vi "AlliGator Check Gate Number in HDF5 File v2.vi"(7 "Gate Names":string[](array[string]), 8 "error in (no error)":errorcluster, 9 "FLI Parameters":T2, 11 "ref in":T1 format="%.0x") -> (0 "error out":errorcluster, 1 "FLI Parameters":T2, 3 "ref":T1 format="%.0x", 4 "Missing Gates?":bool, 6 "Additional Gates?":bool)   [LabVIEW 2021, in "AlliGator HDF5.lvlib"]
doc: "Checks that the gate images stored in the HDF5 file correspond to the description provided by the <B>FLI Parameters</B>.\n\nIf so updates <B># Gates</B> in that structure and sets the corresponding output flags."
uses:
  AlliGator HDF5.lvlib
  Phasor/Phasor Fluorescence Lifetime Parameters v2.ctl
  <vilib>/addons/h5labview2/base/hid_t.ctl
  Arrays/Linear Ramp End Options.ctl
  3b143c5f-f340-4cb5-b493-7761f7e72ec4.vi
  57e33c98-4f83-48b5-b2ca-9a3f9f880677.vi
  <userlib>/_OpenG.lib/array/array.llb/Filter 1D Array (I32)__ogtk.vi
  <vilib>/addons/h5labview2/group/H5G.lvlib
  Arrays/Arrays.lvlib
  <userlib>/_OpenG.lib/array/array.llb/openg_array.lvlib
  Phasor/Phasor.lvlib
panel:
  # "see the AlliGator License on the block diagram (Ctrl+E or Window:Show Block Diagram)"
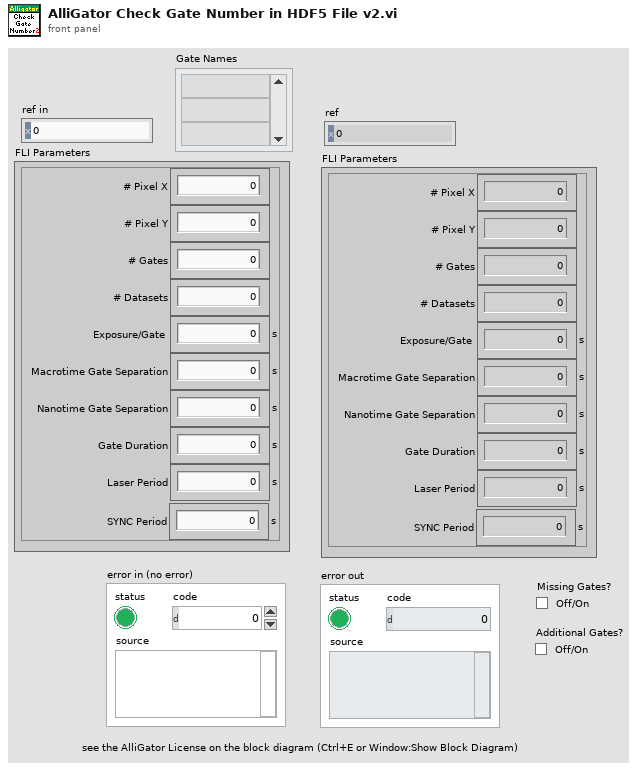
[diagram p1: front panel]
types:
  T1 = typedef "hid_t.ctl" = i64
  T2 = typedef "Phasor.lvlib/Phasor Fluorescence Lifetime Parameters v2.ctl" = cluster{"# Pixel X":i32, "# Pixel Y":i32, "# Gates":i32, "# Datasets":i32, "Exposure/Gate":dbl[unit], "Macrotime Gate Separation":dbl[unit], "Nanotime Gate Separation":dbl[unit], "Gate Duration":dbl[unit], "Laser Period":dbl[unit], "SYNC Period":dbl[unit]}
  T3 = typedef "Arrays.lvlib/Linear Ramp End Options.ctl" = enum16{"Include Min/Exclude Max", "Exclude Min/Include Max", "Include Both Ends", "Exclude Both Ends"}
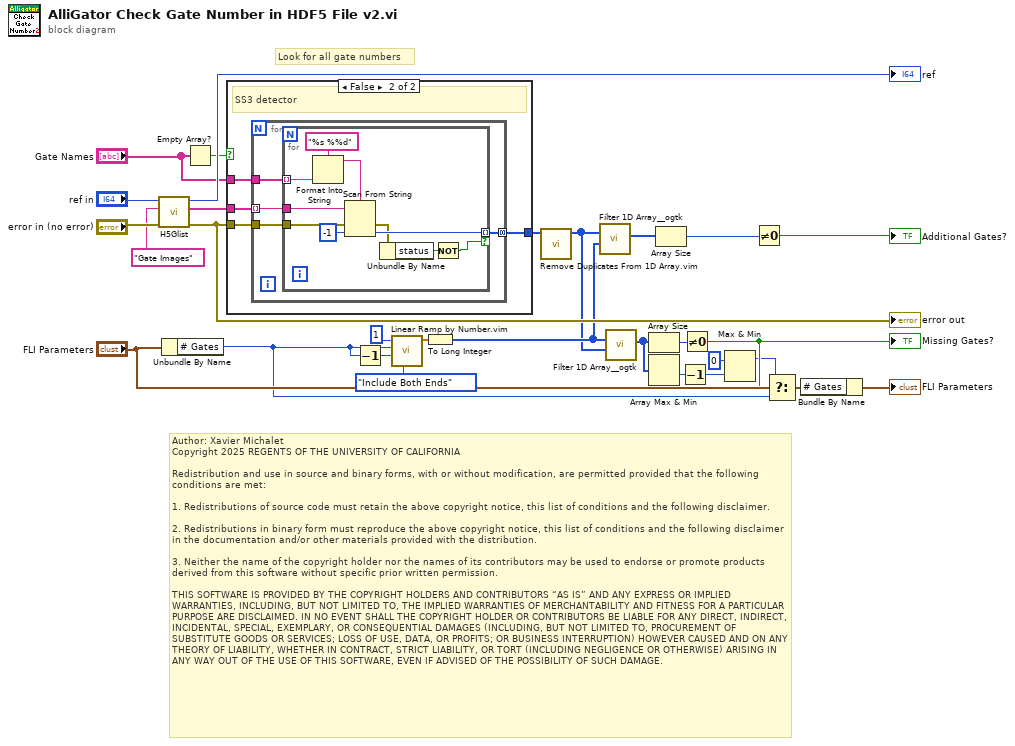
[diagram p0: block diagram]
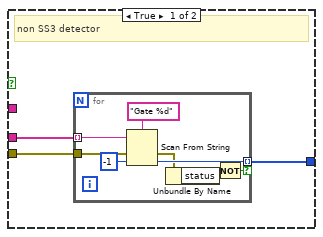
[diagram p2: hidden frame]
diagram:
  # "Author: Xavier Michalet\nCopyright 2025 REGENTS OF THE UNIVERSITY OF CALIFORNIA\n\nRedistribution and use in source and binary forms, with or without modification, are permitted provided that the following conditions are met:\n\n1. Redistributions of source code must retain the above copyright notice, this list of conditions and the following disclaimer.\n\n2. Redistributions in binary form must reproduce the above copyright notice, this list of conditions and the following disclaimer in the documentation and/or other materials provided with the distribution.\n\n3. Neither the name of the copyright holder nor the names of its contributors may be used to endorse or promote products derived from this software without specific prior written permission.\n\nTHIS SOFTWARE IS PROVIDED BY THE COPYRIGHT HOLDERS AND CONTRIBUTORS “AS IS” AND ANY EXPRESS OR IMPLIED WARRANTIES, INCLUDING, BUT NOT LIMITED TO, THE IMPLIED WARRANTIES OF MERCHANTABILITY AND FITNESS FOR A PARTICULAR PURPOSE ARE DISCLAIMED. IN NO EVENT SHALL THE COPYRIGHT HOLDER OR CONTRIBUTORS BE LIABLE FOR ANY DIRECT, INDIRECT, INCIDENTAL, SPECIAL, EXEMPLARY, OR CONSEQUENTIAL DAMAGES (INCLUDING, BUT NOT LIMITED TO, PROCUREMENT OF SUBSTITUTE GOODS OR SERVICES; LOSS OF USE, DATA, OR PROFITS; OR BUSINESS INTERRUPTION) HOWEVER CAUSED AND ON ANY THEORY OF LIABILITY, WHETHER IN CONTRACT, STRICT LIABILITY, OR TORT (INCLUDING NEGLIGENCE OR OTHERWISE) ARISING IN ANY WAY OUT OF THE USE OF THIS SOFTWARE, EVEN IF ADVISED OF THE POSSIBILITY OF SUCH DAMAGE."
  # "Look for all gate numbers"
  n1 = call <vilib>:"H5Glist.vi"("error in (no error)"="error in (no error)", "group (.)"="Gate Images" ("name"), "ref in"="ref in") -> ("error out"=w14:errorcluster, "names"=w23:string[], "ref out"=→"ref":T1)  [unwired: 5 in, 1 out]
  "error out" <- w14
  n2 = Unbundle By Name("FLI Parameters") -> ("# Gates"=w6:i32)
  n3 = Empty Array?(array="Gate Names") -> (empty?=w3:bool)
  n4 = case shown="False" w3 {
    tunnel: w23 -> [w32 w44]
    tunnel: [w31 w43] -> w19
    tunnel: w14 -> [w30 w42]
    tunnel: "Gate Names" -> [_ w41]
    frame True {
      # "non SS3 detector"
      n5 = for {
        tunnel: w32 -> [w39] mode=indexing
        tunnel: w30 -> [w38]
        tunnel: [w37] -> w31 mode=indexing if=w33
        n6 = Scan From String(format string="Gate %d" ("initial string"), input string=w39, error in=w38, default 1=-1 ("default value 1")) -> (error out=w36:errorcluster, output 1=w37:i32)  [unwired: 1 in, 2 out]
        n7 = Unbundle By Name(w36) -> ("status"=w35:bool)
        n8 = Not(x=w35) -> (.not. x?=w33:bool)
      }
    }
    frame False {
      # "SS3 detector"
      n9 = for {
        tunnel: w44 -> [w48] mode=indexing
        tunnel: w42 -> [w47]
        tunnel: [w46] -> w43 mode=concatenating
        tunnel: w41 -> [w45]
        n10 = for {
          tunnel: w48 -> [w58]
          tunnel: w47 -> [w57]
          tunnel: [w56] -> w46 mode=indexing if=w49
          tunnel: w45 -> [w52] mode=indexing
          n11 = Format Into String(format string="%s %%d", w52) -> (resulting string=w50:string)  [unwired: 2 in, 1 out]
          n12 = Scan From String(format string=w50, input string=w58, error in=w57, default 1=-1 ("default value 1")) -> (error out=w55:errorcluster, output 1=w56:i32)  [unwired: 1 in, 2 out]
          n13 = Unbundle By Name(w55) -> ("status"=w54:bool)
          n14 = Not(x=w54) -> (.not. x?=w49:bool)
        }
      }
    }
  }
  n15 = Decrement(x=w6) -> (x-1=w5:i32)
  n16 = call "Linear Ramp by Number.vim"("Options"=Linear_Ramp_End_Options."Include Both Ends", "# Steps (1)"=w5, "End (1)"=w6, "Start (0)"=1) -> ("Ramp"=w18:dbl[])  [unwired: 5 in, 2 out]
  n17 = To Long Integer(number=w18) -> (32bit integer=w4:i32[])
  n18 = call "Remove Duplicates From 1D Array.vim"("array"=w19) -> ("array with duplicates removed"=w1:i32[])  [unwired: 10 in]
  n19 = call-poly <userlib>:"Filter 1D Array__ogtk.vi"("items to filter"=w4, "array"=w1) -> ("filtered array"=w16:i32[])  [unwired: 4 in, 1 out]
  n20 = call-poly <userlib>:"Filter 1D Array__ogtk.vi"("items to filter"=w1, "array"=w4) -> ("filtered array"=w12:i32[])  [unwired: 4 in, 1 out]
  n21 = Array Size(array=w12) -> (size(s)=w20:i32)
  n22 = Array Max & Min(array=w12) -> (min value=w11:i32)  [unwired: 3 out]
  n23 = Array Size(array=w16) -> (size(s)=w17:i32)
  n24 = Decrement(x=w11) -> (x-1=w10:i32)
  n25 = Not Equal To 0?(x=w20) -> (x != 0?=w13:bool)
  "Missing Gates?" <- w13
  n26 = Max & Min(x=0, y=w10) -> (max(x,y)=w8:i32)  [unwired: 1 out]
  n27 = Not Equal To 0?(x=w17) -> (x != 0?=→"Additional Gates?":bool)
  n28 = Select(t=w8, s=w13, f=w6) -> (s? t:f=w7:i32)
  n29 = Bundle By Name(cluster="FLI Parameters", "# Gates"=w7) -> (→"FLI Parameters":T2)
